vi "FTW-Package-Lossy-Multipart-Initialize.vi"(0 "FTW-Message-Lossy In":refnum<class "FTW-Package-Lossy.lvclass">, 5 "Message Parts":string[](array[string]), 11 "error in":errorcluster) -> (4 "FTW-Message-Lossy Out":refnum<class "FTW-Package-Lossy.lvclass">, 6 "overflow?":bool, 15 "error out":errorcluster)   [LabVIEW 2013, in "FTW-Package-Lossy.lvclass"]
uses:
  FTW-Package-Lossy.lvclass
  FTW-Package-Lossy.lvclass/FTW-Package-Lossy.ctl
panel:
  # "Inputs"
  # "Outputs"
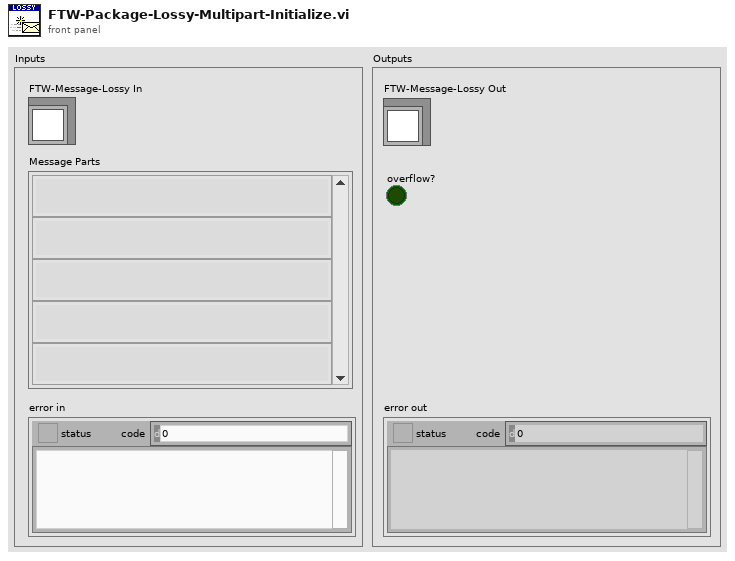
[diagram p1: front panel]
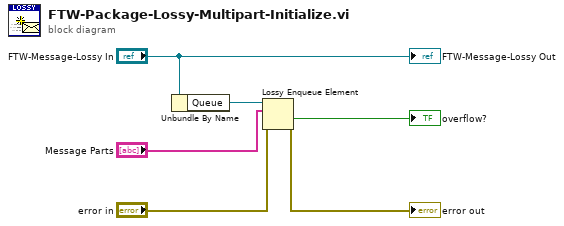
[diagram p0: block diagram]
diagram:
  n1 = Unbundle By Name("FTW-Message-Lossy In") -> ("Queue"=w1:refnum<queue>)
  n2 = Lossy Enqueue Element(queue=w1, element="Message Parts", error in (no error)="error in") -> (overflow?=→"overflow?":bool, error out=→"error out":errorcluster)  [unwired: 2 out]
  "FTW-Message-Lossy Out" <- "FTW-Message-Lossy In"
